vi "Create and Test Single Topology.vi"() -> ()   [LabVIEW 2017]
uses:
  <vilib>/SLSC_Switch/Path Capability.ctl
  Slot Module Selection.ctl
  <vilib>/SLSC_Switch/SLSC Switch.lvlib
panel:
  in  "Base Topology Path":path=path "C:/github/SLSC-Switch-Topology-Generator/source/json files/SET-2010 Base.json"
  in  "error in":errorcluster
  out "error out":errorcluster
  in  "Output Directory":path=path "C:/github/SLSC-Switch-Topology-Generator/output"
  in  "Slot 2 Module Selection":T1
  in  "Slot 1 Module Selection":T1
  out "Array":T3(array[cluster]) {"path capability" items=["Path Available"=1, "Path Exists"=2, "Path Unsupported"=3, "Resource in Use"=4, "Source Conflict"=5, "Channel Not Available"=6]; "path capability" items=["Path Available"=1, "Path Exists"=2, "Path Unsupported"=3, "Resource in Use"=4, "Source Conflict"=5, "Channel Not Available"=6]}
  # "Source"
  # "Destination"
  # "Base"
  # "Generated"
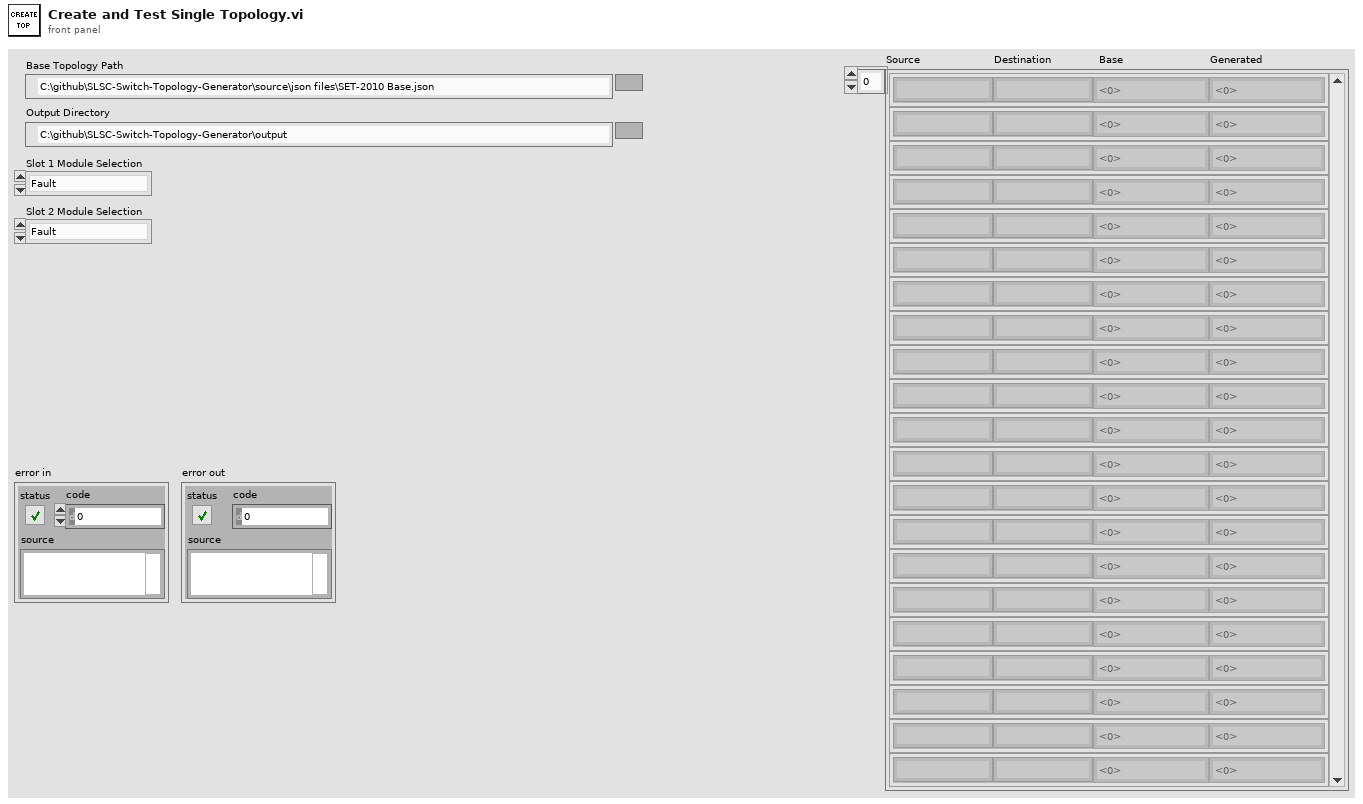
[diagram p1: front panel]
types:
  T1 = typedef "Slot Module Selection.ctl" = enum16{"Fault", "Instrument", "Empty"}
  T2 = typedef "SLSC Switch.lvlib/Path Capability.ctl" = i32
  T3 = cluster{string, string, "path capability":T2, "path capability":T2}[]
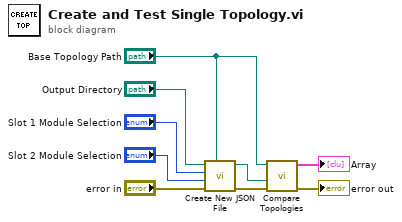
[diagram p0: block diagram]
diagram:
  n1 = call "Create New JSON File.vi"("Source Base JSON File"="Base Topology Path", "error in"="error in", "Slot 2 Module Selection"="Slot 2 Module Selection", "Slot 1 Module Selection"="Slot 1 Module Selection", "Output Directory"="Output Directory") -> ("error out"=w4:errorcluster, "path out"=w2:path)  [unwired: 5 in]
  n2 = call "Compare Topologies.vi"("error in (no error)"=w4, "Modified Base Topology"=w2, "Base Topology"="Base Topology Path") -> ("error out"=→"error out":errorcluster, "Differences"=→"Array":T3)  [unwired: 7 in]
